vi "USRP Dummy_v0 (FPGA).vi"() -> ()   [LabVIEW 2016]
uses:
  <instrlib>/_niInstr/Register Bus/v1/FPGA/Public/Read Cmd Data.ctl
  <vilib>/Platform/TimedLoop/XDataNode/timing_clust.ctl
  <vilib>/Platform/TimedLoop/XDataNode/nitl_modes.ctl
  <vilib>/Platform/TimedLoop/XDataNode/wakeup.ctl
  <vilib>/rvi/Emulation/niFpgaSctlEmulationGetInTimedLoop.vi
  <vilib>/rvi/Emulation/niFpgaEmulationReportErrorSimple.vi
  <vilib>/rvi/Emulation/niFpgaGetClockAttributes.vi
  <vilib>/rvi/Emulation/niFpgaCriticalErrorInLSC.vi
  <vilib>/rvi/eio/common/nirviEmuTemplateMethod_errors.vi
  <vilib>/rvi/interface/RandomDataEmulation/niFpgaRandomDataHandleErrors.vi
  <vilib>/Platform/TimedLoop/XDataNode/XDataNode.xnode
  <vilib>/eio/EIONode/EIONode.xnode
  <vilib>/rvi/DataTransferAndStorage/Container/XNode/niFpgaContainer.xnode
  <vilib>/rvi/interface/RandomDataEmulation/nirviRandomDataFpgaReadWriteTemplate.vi
  <vilib>/Platform/TimedLoop/XDataNode/XDNodeRunTimeDep.lvlib
  <instrlib>/_niInstr/Register Bus/v1/FPGA/niInstr Register Bus v1 FPGA.lvlib
  <instrlib>/niUsrpRio/Config/v1/FPGA/niUsrpRio Config v1 FPGA.lvlib
  <instrlib>/_niInstr/Basic Elements/v1/FPGA/niInstr Basic Elements v1 FPGA.lvlib
panel:
  out "Random Number":u8
  in  "Flush FIFO?":bool
  in  "Stop Transfer?":bool
  out "Min Space Available":u32
  out "Space Available":u32
  out "FPGA FIFO Depth":u32
  in  "Reset FPGA Count?":bool
  out "Send Status?":bool
  out "Samples Left to Write":u64
  in  "Number of Samples":u64
  in  "reg.host read.go rcvd 0":bool
  out "reg.notify host.go 0":bool
  in  "reg.notify host.go rcvd 0":bool
  out "reg.host read.data 0":T1
  in  "reg.reset 0":bool
  in  "RF 0/Rx/Enable":bool
  in  "RF 0/Tx/Enable":bool
  in  "RF 1/Rx/Enable":bool
  in  "RF 1/Tx/Enable":bool
  out "FPGA Transfer Count":u64
  in  "Start Transfer?":bool
  in  "Reset Timeouts?":bool
  out "Timeout Count":u64
  out "Sticky Timeout?":bool
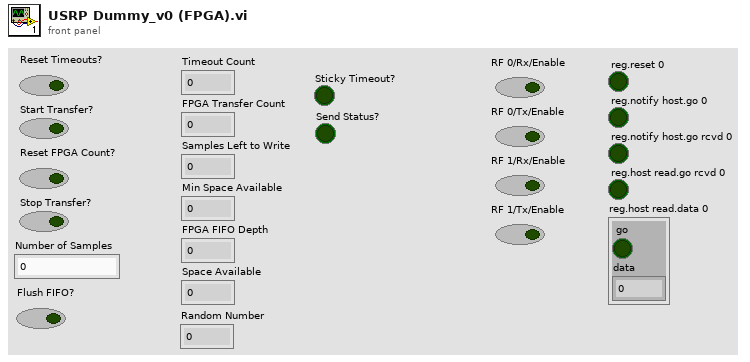
[diagram p1: front panel]
types:
  T1 = typedef "niInstr Register Bus v1 FPGA.lvlib/Read Cmd Data.ctl" = cluster{"go":bool, "data":u32}
  T2 = typedef "XDNodeRunTimeDep.lvlib/timing_clust.ctl" = cluster{"Expected End [f-1]":u64, "Actual End [f-1]":u64, "Finished Late? [f-1]":bool, "Expected End [i-1]":u64, "Actual End [i-1]":u64, "Finished Late? [i-1]":bool, "Expected Start [i]":u64, "Actual Start [i]":u64, "Expected Start [f]":u64, "Actual Start [f]":u64, "Source Name":string, "Structure Name":string, "Period":i64, "Deadline":i64, "Offset":i64, "Start":i64, "Priority":i32, "Timeout":i32, "Mode":T3, "Wakeup Reason":T4, "Error":errorcluster, "Source Type":string, "Secondary Source Type":string, "Global End Time":u64, "Global Start Time":u64, "Frame Duration":u64, "Iteration Duration":u64, "Assigned CPU":i32, "I/O Scan Engine Mode":u32}
  T3 = typedef "XDNodeRunTimeDep.lvlib/nitl_modes.ctl" = enum32{"No Change", "Process missed periods, maintain original phase", "Discard missed periods, maintain original phase", "Process missed periods, ignore original phase", "Discard missed periods, ignore original phase"}
  T4 = typedef "XDNodeRunTimeDep.lvlib/wakeup.ctl" = enum32{"Normal", "Aborted", "Asynchronous wakeup", "Timing source error", "Timed loop error", "Timeout"}
  T5 = cluster{"DAC FIFO Reset":refnum<k21>, "RF 0 Rx Swap IQ":refnum<k21>, "RF 0 Rx Negate I":refnum<k21>, "RF 0 Rx Negate Q":refnum<k21>, "RF 0 Rx Data Valid":refnum<k21>, "RF 0 Rx Data Ever Invalid":refnum<k21>, "clear RF 0 Rx Data Ever Invalid":refnum<k21>, "RF 0 Tx Swap IQ":refnum<k21>, "RF 0 Tx Negate I":refnum<k21>, "RF 0 Tx Negate Q":refnum<k21>, "RF 1 Rx Swap IQ":refnum<k21>, "RF 1 Rx Negate I":refnum<k21>, "RF 1 Rx Negate Q":refnum<k21>, "RF 1 Rx Data Valid":refnum<k21>, "RF 1 Rx Data Ever Invalid":refnum<k21>, "clear RF 1 Rx Data Ever Invalid":refnum<k21>, "RF 1 Tx Swap IQ":refnum<k21>, "RF 1 Tx Negate I":refnum<k21>, "RF 1 Tx Negate Q":refnum<k21>}
  T6 = typedef "niUsrpRio Synchronization v1 FPGA.lvlib/Resources.ctl" = cluster{"master":refnum<k21>, "meas.enable":refnum<k21>, "meas.ready":refnum<k21>, "meas.reset":refnum<k21>, "meas.arm":refnum<k21>, "meas.valid":refnum<k21>, "meas.value":refnum<k21>, "meas.oversample factor":refnum<k21>, "cptr":refnum<k21>, "cptr.adjust":refnum<k21>, "cptr.period":refnum<k21>}
  T7 = typedef "niUsrpRio Time v1 FPGA.lvlib/Time Resources.ctl" = cluster{"reset":refnum<k21>, "time":refnum<k21>, "time.previous cptr":refnum<k21>, "new time":refnum<k21>, "new time.when":refnum<k21>, "new time.set":refnum<k21>, "which edge of ref":refnum<k21>, "pps source":refnum<k21>, "internal pps period":refnum<k21>}
  T8 = typedef "niUsrpRio Time v1 FPGA.lvlib/Future Event Resources.ctl" = cluster{"reset":refnum<k21>, "future event.time":refnum<k21>, "future event.ready":refnum<k21>, "future event.set":refnum<k21>, "future event.clear":refnum<k21>, "future event.set in past":refnum<k21>}
  T9 = cluster{"time.resources":T7, "future event.resources":T8, "future event.resources":T8, "future event.resources":T8}
  T10 = typedef "niInstr Register Bus v1 FPGA.lvlib/Register Instruction.ctl" = cluster{"subsystem":u8, "address":u16, "data":u32, "valid":bool, "read":bool}
  T11 = typedef "niInstr Register Bus v1 FPGA.lvlib/Read Completion.ctl" = cluster{"data":u32, "valid":bool}
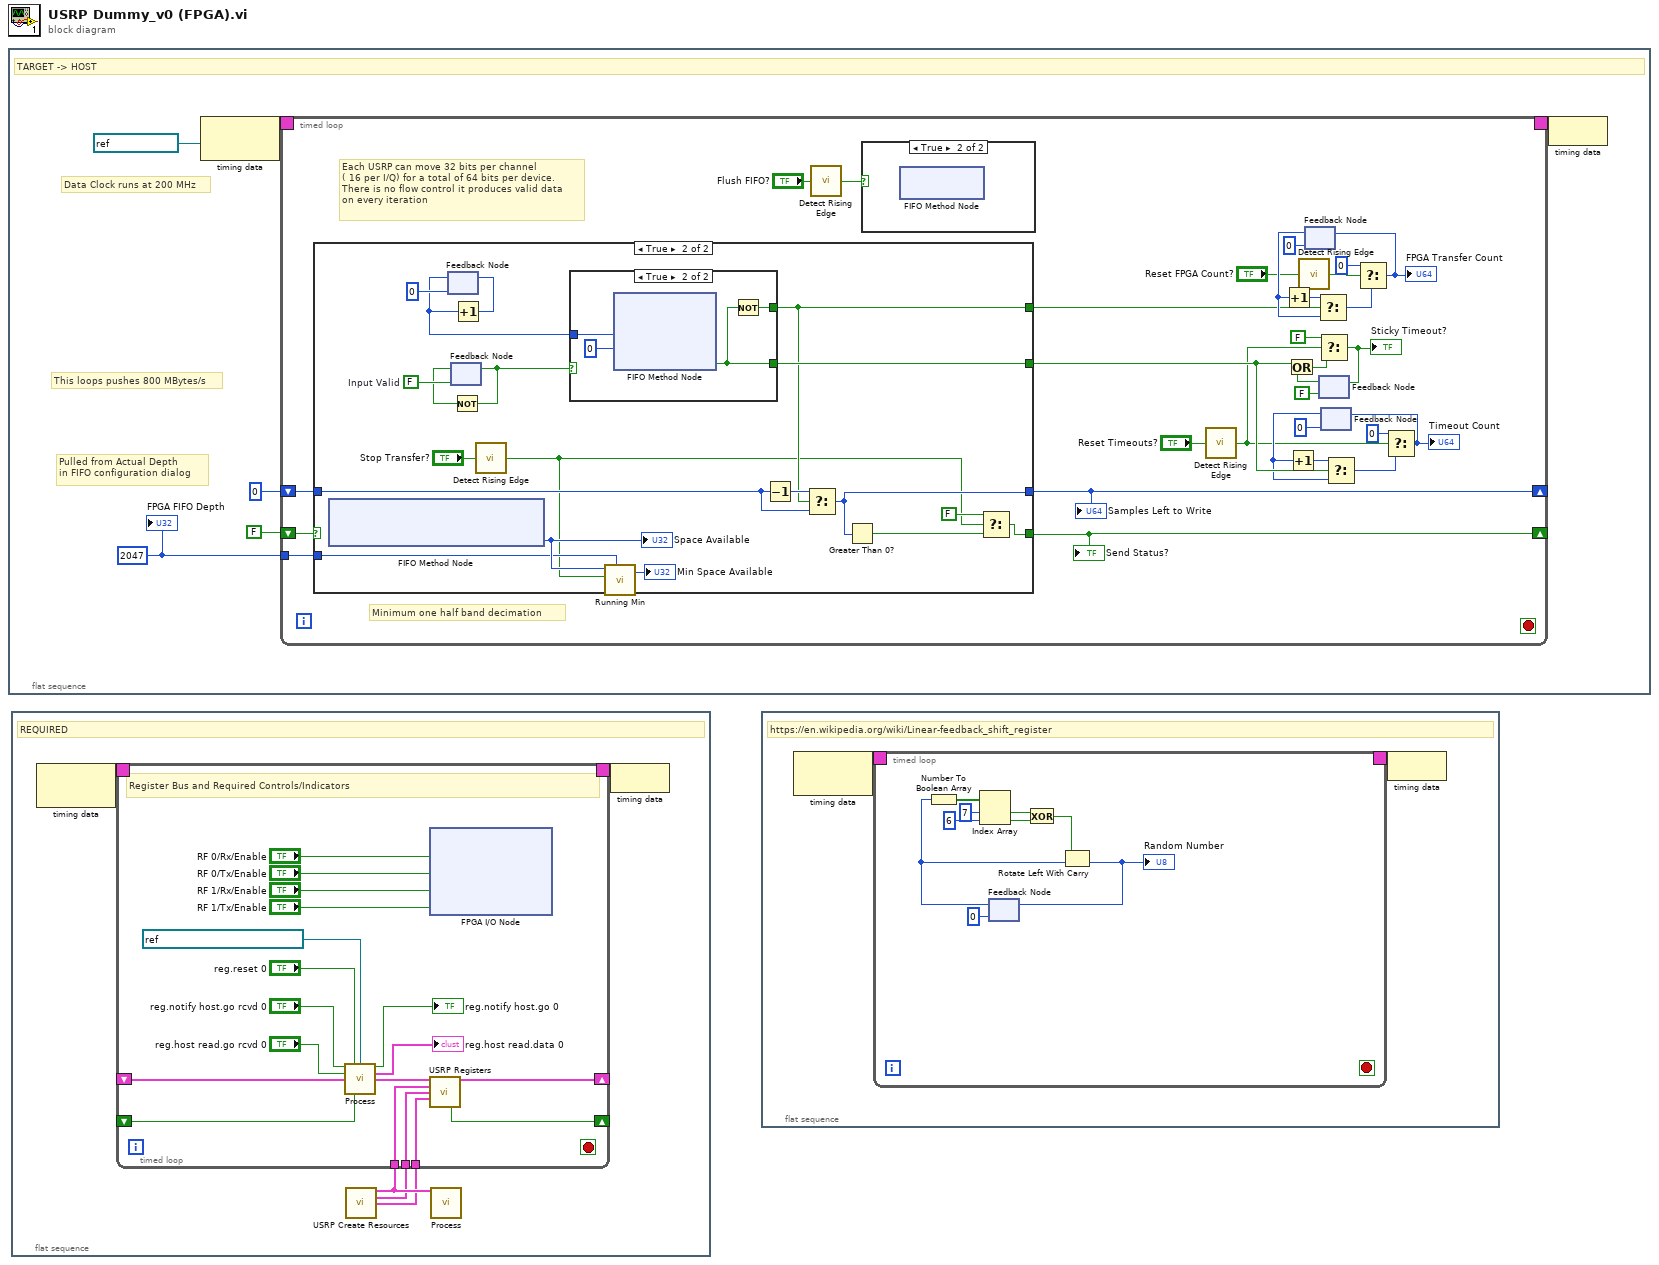
[diagram p0: block diagram]
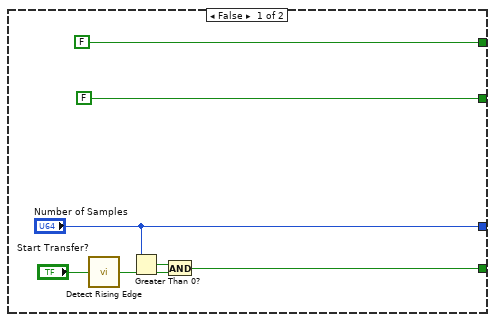
[diagram p3: hidden frame]
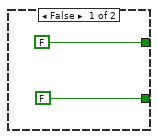
[diagram p4: hidden frame]
diagram:
  n1 = flat-sequence {
    frame #0 {
      w1 = u32 2047 ("FPGA FIFO Depth")
      # "Pulled from Actual Depth\nin FIFO configuration dialog"
      # "This loops pushes 800 MBytes/s"
      # "Data Clock runs at 200 MHz"
      # "TARGET -> HOST"
      n2 = node-c288(refnum<k21> "Data Clock" ("Source Name")) -> (w6:T2)
      n3 = timed-loop {
        timing: w6 -> [_]
        timing-out: [_] -> w5
        shift-right: [w25] -> _
        shift-left: FALSE ("send data?") -> [w24]
        shift-right: [w22] -> _
        shift-left: u64 0 ("samples to write") -> [w23]
        tunnel: w1 -> [w13]
        stop <- _ stop-if-true
        # "Each USRP can move 32 bits per channel\n( 16 per I/Q) for a total of 64 bits per device.\nThere is no flow control it produces valid data\non every iteration"
        # "Minimum one half band decimation"
        n4 = case shown="True" w24 {
          tunnel: [FALSE ("Timed Out?") w48] -> w27
          tunnel: [FALSE ("Timed Out?") w50] -> w26
          tunnel: [w39 w53] -> w25
          tunnel: w23 -> [_ w60]
          tunnel: ["Number of Samples" w61] -> w22
          tunnel: w13 -> [_ w58]
          frame False {
            n5 = call <instrlib>:"Detect Rising Edge.vi"("signal"="Start Transfer?") -> ("edge detected"=w40:bool)  [unwired: 14 in]
            n6 = Greater Than 0?(x="Number of Samples") -> (x > 0?=w38:bool)
            n7 = And(x=w38, y=w40) -> (x .and. y?=w39:bool)
          }
          frame True {
            w52 = FALSE  # Input Valid
            n8 = xnode ("FIFO Method Node")() -> ("Number of Elements to Write"=w59:u32)  [unwired: 1 in, 1 out]
            "Space Available" <- w59
            n9 = feedback #1(u64 0) -> (w44:u64)
            n10 = feedback #2(w52) -> (w51:bool)
            n11 = Not(x=w51) -> (.not. x?=w49:bool)
            n12 = feedback-in #2(w49) -> ()
            n13 = Increment(x=w44) -> (x+1=w46:u64)
            n14 = feedback-in #1(w46) -> ()
            n15 = call <instrlib>:"Detect Rising Edge.vi"("signal"="Stop Transfer?") -> ("edge detected"=w45:bool)  [unwired: 14 in]
            n16 = case shown="True" w49 {
              tunnel: w44 -> [_ w68]
              tunnel: [FALSE ("Timed Out?") w67] -> w50
              tunnel: [FALSE ("Timed Out?") w66] -> w48
              frame False {
              }
              frame True {
                n17 = xnode ("FIFO Method Node")("Element"=w68, "Timeout"=0) -> ("Timed Out?"=w67:bool)  [unwired: 1 in, 1 out]
                n18 = Not(x=w67) -> (.not. x?=w66:bool)
              }
            }
            n19 = call "Running Min.vi"("Starting Min"=w58, "Reset"=w45, "Next Value"=w59) -> ("Running Min"=→"Min Space Available":u32)  [unwired: 4 in]
            n20 = Decrement(x=w60) -> (x-1=w62:u64)
            n21 = Select(t=w62, s=w48, f=w60) -> (s? t:f=w61:u64)
            n22 = Greater Than 0?(x=w61) -> (x > 0?=w54:bool)
            n23 = Select(t=FALSE, s=w45, f=w54) -> (s? t:f=w53:bool)
          }
        }
        "Samples Left to Write" <- w22
        "Send Status?" <- w25
        n24 = call <instrlib>:"Detect Rising Edge.vi"("signal"="Flush FIFO?") -> ("edge detected"=w7:bool)  [unwired: 14 in]
        n25 = case shown="True" w7 {
          frame False {
          }
          frame True {
            n26 = xnode ("FIFO Method Node")() -> ()  [unwired: 1 in, 1 out]
          }
        }
        n27 = call <instrlib>:"Detect Rising Edge.vi"("signal"="Reset Timeouts?") -> ("edge detected"=w12:bool)  [unwired: 14 in]
        n28 = call <instrlib>:"Detect Rising Edge.vi"("signal"="Reset FPGA Count?") -> ("edge detected"=w14:bool)  [unwired: 14 in]
        n29 = feedback #3(u64 0) -> (w29:u64)
        n30 = Increment(x=w29) -> (x+1=w28:u64)
        n31 = Select(t=w28, s=w27, f=w29) -> (s? t:f=w17:u64)
        n32 = feedback #4(FALSE) -> (w32:bool)
        n33 = Or(x=w26, y=w32) -> (x .or. y?=w11:bool)
        n34 = Select(t=FALSE, s=w12, f=w11) -> (s? t:f=w10:bool)
        "Sticky Timeout?" <- w10
        n35 = feedback-in #4(w10) -> ()
        n36 = feedback #5(u64 0) -> (w21:u64)
        n37 = Increment(x=w21) -> (x+1=w20:u64)
        n38 = Select(t=w20, s=w26, f=w21) -> (s? t:f=w35:u64)
        n39 = Select(t=u64 0, s=w14, f=w17) -> (s? t:f=w16:u64)
        "FPGA Transfer Count" <- w16
        n40 = feedback-in #3(w16) -> ()
        n41 = Select(t=u64 0, s=w12, f=w35) -> (s? t:f=w34:u64)
        "Timeout Count" <- w34
        n42 = feedback-in #5(w34) -> ()
      }
      n43 = node-c288(w5) -> ()
      "FPGA FIFO Depth" <- w1
    }
  }
  n44 = flat-sequence {
    frame #0 {
      # "REQUIRED"
      n45 = node-c288() -> (w79:T2)  [unwired: 1 in]
      n46 = call "USRP Create Resources.vi"() -> ("config.resources"=w77:T5, "sync.resources"=w76:T6, "time.resources"=w75:T9)  [unwired: 13 in]
      n47 = timed-loop "Register Bus and Required Controls/Indicators" {
        timing: w79 -> [_]
        timing-out: [_] -> w78
        shift-right: [w94] -> _
        shift-left: _ -> [w93]
        shift-right: [w88] -> _
        shift-left: _ -> [w92]
        tunnel: w77 -> [w86]
        tunnel: w76 -> [w85]
        tunnel: w75 -> [w84]
        stop <- _ stop-if-true
        # "Register Bus and Required Controls/Indicators"
        n48 = call <instrlib>:"Process.vi"("reg.notify host.go rcvd"="reg.notify host.go rcvd 0", "reg.reset"="reg.reset 0", "reg.host instruction fifo"=refnum<k21> "reg.host instruction fifo 0", "reg.host read.go rcvd"="reg.host read.go rcvd 0", "read completion"=w93, "ready for output"=w92) -> ("reg.notify host.go"=→"reg.notify host.go 0":bool, "reg.host read.data"=→"reg.host read.data 0":T1, "register instruction"=w87:T10)  [unwired: 7 in]
        n49 = xnode ("FPGA I/O Node")("RF 0/Rx/Enable"="RF 0/Rx/Enable", "RF 0/Tx/Enable"="RF 0/Tx/Enable", "RF 1/Rx/Enable"="RF 1/Rx/Enable", "RF 1/Tx/Enable"="RF 1/Tx/Enable") -> ()  [unwired: 4 in, 4 out]
        n50 = call "USRP Registers.vi"("register instruction"=w87, "config.resources"=w86, "sync.resources"=w85, "time.resources"=w84) -> ("read completion out"=w94:T11, "ready for input"=w88:bool)  [unwired: 10 in]
      }
      n51 = call <instrlib>:"Process.vi"("resources"=w77) -> ()  [unwired: 15 in]
      n52 = node-c288(w78) -> ()
    }
  }
  n53 = flat-sequence {
    frame #0 {
      # "https://en.wikipedia.org/wiki/Linear-feedback_shift_register"
      n54 = node-c288() -> (w103:T2)  [unwired: 1 in]
      n55 = timed-loop {
        timing: w103 -> [_]
        timing-out: [_] -> w102
        stop <- _ stop-if-true
        n56 = feedback #6(u8 0) -> (w106:u8)
        n57 = Number To Boolean Array(number=w106) -> (Boolean array=w112:bool[])
        n58 = Index Array(array=w112, index #1=7 ("index"), index #2=6 ("index")) -> (element #1=w108:bool, element #2=w107:bool)
        n59 = Exclusive Or(1:w107, 2:w108) -> (0:w105:bool)
        n60 = Rotate Left With Carry(2:w106, 3:w105) -> (0:w104:u8)  [unwired: 1 out]
        "Random Number" <- w104
        n61 = feedback-in #6(w104) -> ()
      }
      n62 = node-c288(w102) -> ()
    }
  }
